vi "Compra.vi"(8 "error in (no error)":errorcluster, 10 "Producto":string[](array[string]), 11 "UI Actor in":refnum<class "UI Actor.lvclass">) -> (0 "error out":errorcluster, 3 "UI Actor out":refnum<class "UI Actor.lvclass">)   [LabVIEW 2020, in "UI Actor.lvlib" / "UI Actor.lvclass"]
uses:
  UI Actor.lvclass
  UI Actor.lvclass/UI Actor.ctl
  MSG Messages/Update msg Msg/Update msg Msg.lvclass/Update msg Msg.ctl
  <vilib>/ActorFramework/Message Enqueuer/Message Enqueuer.lvclass/Message Enqueuer.ctl
  LHL Actor Messages/Inventario Msg/Inventario Msg.lvclass/Inventario Msg.ctl
  <vilib>/ActorFramework/Message Enqueuer/Init from Existing Queue.vi
  <vilib>/ActorFramework/Message Enqueuer/Enqueue.vi
  MSG Messages/Update msg Msg/Update msg Msg.lvclass
  C:/Program Files/National Instruments/LabVIEW 2020/vi.lib/ActorFramework/Message/Message.lvclass
  LHL Actor Messages/Inventario Msg/Inventario Msg.lvclass
  <vilib>/ActorFramework/Message Priority Queue/Priority Enqueue.vi
  <vilib>/ActorFramework/Message Enqueuer/Message Enqueuer.lvclass
  <vilib>/ActorFramework/Actor/Actor.lvclass
  C:/Program Files/National Instruments/LabVIEW 2020/vi.lib/ActorFramework/Actor/Actor.lvclass
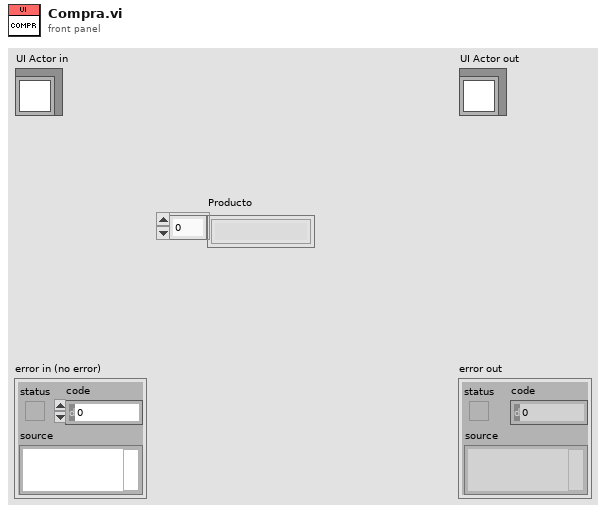
[diagram p1: front panel]
types:
  T1 = enum16{"La Hogaza de Lui", "MiniSuper Doña Rata"}
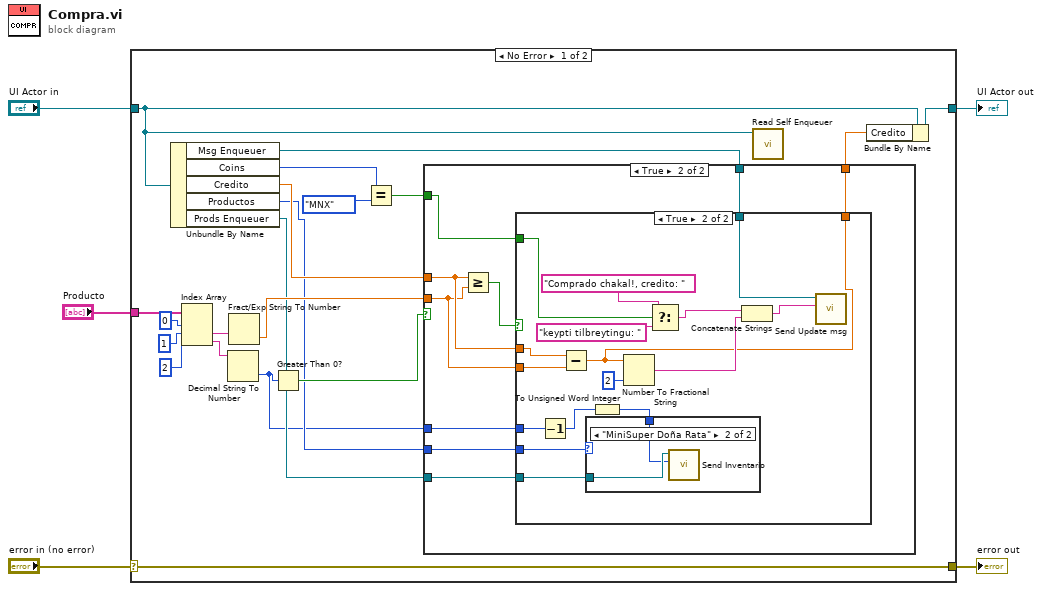
[diagram p0: block diagram]
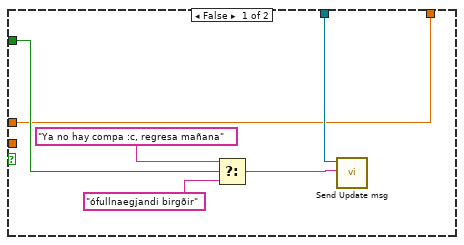
[diagram p2: hidden frame]
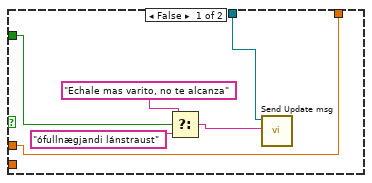
[diagram p3: hidden frame]
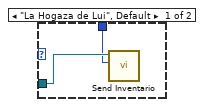
[diagram p4: hidden frame]
diagram:
  n1 = case shown="No Error" "error in (no error)" {
    selector: "error in (no error)" -> [w25 w68]
    tunnel: [w25 w68] -> w4
    tunnel: [w10 w67] -> w2
    tunnel: "UI Actor in" -> [w11 w67]
    tunnel: "Producto" -> [w22 _]
    frame No Error {
      n2 = Unbundle By Name(w11) -> ("Msg Enqueuer"=w15:refnum<class "Message Enqueuer.lvclass">, "Coins"=w24:enum16{"MNX", "Corona Islandesa"}, "Credito"=w12:dbl, "Productos"=w7:T1, "Prods Enqueuer"=w8:refnum<class "Message Enqueuer.lvclass">)
      n3 = Index Array(array=w22, index #1=0 ("index"), index #2=1 ("index"), index #3=2 ("index")) -> (element #2=w14:string, element #3=w18:string)  [unwired: 1 out]
      n4 = Decimal String To Number(string=w18) -> (number=w6:i32)  [unwired: 2 in, 1 out]
      n5 = Fract/Exp String To Number(string=w14) -> (number=w13:dbl)  [unwired: 3 in, 1 out]
      n6 = Greater Than 0?(x=w6) -> (x > 0?=w17:bool)
      n7 = Equal?(x=w24, y=enum16{"MNX", "Corona Islandesa"}."MNX") -> (x = y?=w16:bool)
      n8 = case shown="True" w17 {
        tunnel: w16 -> [w31 w39]
        tunnel: w15 -> [w28 w36]
        tunnel: w13 -> [_ w37]
        tunnel: w12 -> [w26 w38]
        tunnel: [w26 w35] -> w9
        tunnel: w8 -> [_ w33]
        tunnel: w7 -> [_ w34]
        tunnel: w6 -> [_ w32]
        frame False {
          n9 = Select(t="Ya no hay compa :c, regresa mañana", s=w31, f="ófullnaegjandi birgðir") -> (s? t:f=w27:string)
          n10 = call "Send Update msg.vi"("Update msg"=w27, "Message Enqueuer"=w28) -> ()  [unwired: 8 in, 2 out]
        }
        frame True {
          n11 = Greater Or Equal?(x=w38, y=w37) -> (x >= y?=w40:bool)
          n12 = case shown="True" w40 {
            tunnel: w39 -> [w44 w62]
            tunnel: w38 -> [w41 w60]
            tunnel: w37 -> [_ w59]
            tunnel: w36 -> [w42 w54]
            tunnel: [w41 w52] -> w35
            tunnel: w34 -> [_ w51]
            tunnel: w33 -> [_ w50]
            tunnel: w32 -> [_ w49]
            frame False {
              n13 = Select(t="Echale mas varito, no te alcanza", s=w44, f="ófullnægjandi lánstraust") -> (s? t:f=w43:string)
              n14 = call "Send Update msg.vi"("Update msg"=w43, "Message Enqueuer"=w42) -> ()  [unwired: 8 in, 2 out]
            }
            frame True {
              n15 = Decrement(x=w49) -> (x-1=w48:i32)
              n16 = Subtract(x=w60, y=w59) -> (x-y=w52:dbl)
              n17 = To Unsigned Word Integer(number=w48) -> (unsigned 16bit integer=w47:u16)
              n18 = case shown="\"MiniSuper Doña Rata\"" w51 {
                tunnel: w50 -> [w64 w66]
                tunnel: w47 -> [w63 w65]
                frame "La Hogaza de Lui", Default {
                  n19 = call "Send Inventario.vi"("Numeric"=w63, "Message Enqueuer"=w64) -> ()  [unwired: 8 in, 2 out]
                }
                frame "MiniSuper Doña Rata" {
                  n20 = call "Send Inventario.vi"("Inventario"=w65, "Message Enqueuer"=w66) -> ()  [unwired: 8 in, 2 out]
                }
              }
              n21 = Number To Fractional String(number=w52, precision (6)=i16 2) -> (F-format string=w57:string)  [unwired: 2 in]
              n22 = Select(t="Comprado chakal!, credito: ", s=w62, f="keypti tilbreytingu: ") -> (s? t:f=w55:string)
              n23 = Concatenate Strings(w55, w57) -> (w53:string)
              n24 = call "Send Update msg.vi"("Update msg"=w53, "Message Enqueuer"=w54) -> ()  [unwired: 8 in, 2 out]
            }
          }
        }
      }
      n25 = call <vilib>:"Read Self Enqueuer.vi"("Actor"=w11) -> ()  [unwired: 10 in, 1 out]
      n26 = Bundle By Name(cluster=w11, "Credito"=w9) -> (w10:refnum<class "UI Actor.lvclass">)
    }
    frame Error {
    }
  }
  "error out" <- w4
  "UI Actor out" <- w2
